vi "Read Exporter.vi"(9 "Selection":string, 11 "UIManager in":refnum<class "UIManager.lvclass">) -> (1 "Parameters":string, 2 "IExporter.lvclass":refnum<class "IExporter.lvclass">, 3 "UIManager out":refnum<class "UIManager.lvclass">, 4 "found?":bool)   [LabVIEW 2020, in "DependencyInspector.lvlib" / "UIManager.lvclass"]
uses:
  UIManager.lvclass
  ExtensionInterfaces/IExporter/IExporter.lvclass
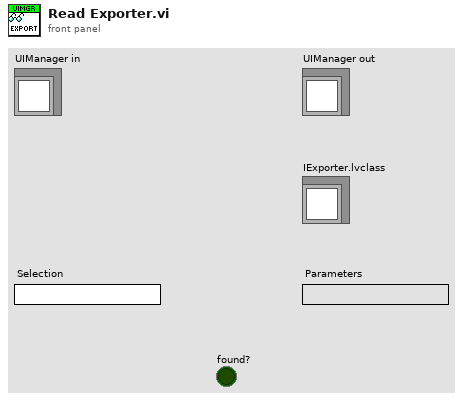
[diagram p1: front panel]
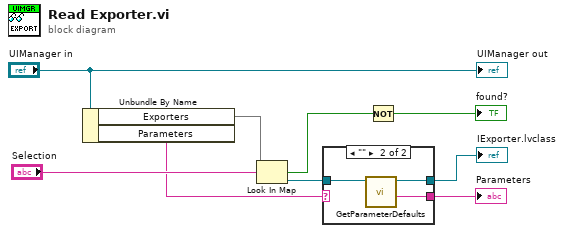
[diagram p0: block diagram]
diagram:
  n1 = Unbundle By Name("UIManager in") -> ("Exporters"=w8:map{string, refnum<class "IExporter.lvclass">}, "Parameters"=w4:string)
  n2 = Look In Map(map=w8, key="Selection") -> (key not found?=w6:bool, value=w3:refnum<class "IExporter.lvclass">)  [unwired: 1 in]
  n3 = case shown="\"\"" w4 {
    selector: w4 -> [w11 _]
    tunnel: [w11 w13] -> w1
    tunnel: w3 -> [w10 w14]
    tunnel: [w10 w12] -> w2
    frame Default {
    }
    frame "" {
      n4 = call-dynamic "GetParameterDefaults.vi"("IExporter in"=w14) -> ("Parameter defaults"=w13:string, "IExporter out"=w12:refnum<class "IExporter.lvclass">)  [unwired: 8 in, 1 out]
    }
  }
  "IExporter.lvclass" <- w2
  "Parameters" <- w1
  n5 = Not(x=w6) -> (.not. x?=→"found?":bool)
  "UIManager out" <- "UIManager in"
